vi "KE487_Test.vi"(8 "error in (no error)":errorcluster, 11 "KE487 in":refnum<class "KE487.lvclass">) -> (0 "error out":errorcluster, 3 "KE487 out":refnum<class "KE487.lvclass">)   [LabVIEW 2013, in "KE487.lvclass"]
uses:
  KE487.lvclass
  <vilib>/Platform/TimedLoop/XDataNode/timing_clust.ctl
  <vilib>/Platform/TimedLoop/XDataNode/nitl_modes.ctl
  <vilib>/Platform/TimedLoop/XDataNode/wakeup.ctl
  InstrumentSetup.vi
  <vilib>/platform/TimedLoop/XDataNode/XDataNode.xnode
  <vilib>/Platform/TimedLoop/XDataNode/XDNodeRunTimeDep.lvlib
  InstrControl.lvclass
panel:
  out "Current [nA]":dbl
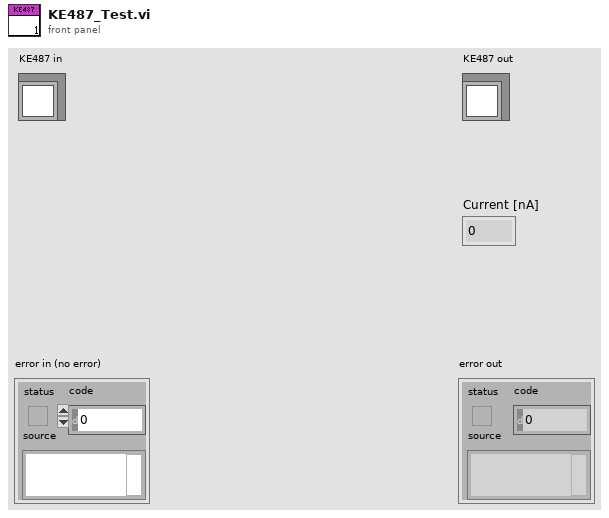
[diagram p1: front panel]
types:
  T1 = cluster{"KE 2410":cluster{"Instrument name":string, "address":refnum<visa-resource-name>, "Instrument type":u16}, "KE 6517":cluster{"Instrument name":string, "address":refnum<visa-resource-name>, "Instrument type":u16}, "KE 487":cluster{"Instrument name":string, "address":refnum<visa-resource-name>, "Instrument type":u16}, "KE 236":cluster{"Instrument name":string, "address":refnum<visa-resource-name>, "Instrument type":u16}, "WK 6440B":cluster{"Instrument name":string, "address":refnum<visa-resource-name>, "Instrument type":u16}, "WK 6425":cluster{"Instrument name":string, "address":refnum<visa-resource-name>, "Instrument type":u16}, "Pickering Matrix":cluster{"Instrument name":string, "address":refnum<visa-resource-name>, "Instrument type":u16}, "KE 2000":cluster{"Instrument name":string, "address":refnum<visa-resource-name>, "Instrument type":u16}, "KE3706A Switching":cluster{"Instrument name":string, "address":refnum<visa-resource-name>, "Instrument type":u16}}
  T2 = cluster{"Compliance":u16, "Range:":u16, "KE487":refnum<class "KE487.lvclass">}
  T3 = typedef "XDNodeRunTimeDep.lvlib/timing_clust.ctl" = cluster{"Expected End [f-1]":u64, "Actual End [f-1]":u64, "Finished Late? [f-1]":bool, "Expected End [i-1]":u64, "Actual End [i-1]":u64, "Finished Late? [i-1]":bool, "Expected Start [i]":u64, "Actual Start [i]":u64, "Expected Start [f]":u64, "Actual Start [f]":u64, "Source Name":string, "Structure Name":string, "Period":i64, "Deadline":i64, "Offset":i64, "Start":i64, "Priority":i32, "Timeout":i32, "Mode":T4, "Wakeup Reason":T5, "Error":errorcluster, "Source Type":string, "Secondary Source Type":string, "Global End Time":u64, "Global Start Time":u64, "Frame Duration":u64, "Iteration Duration":u64, "Assigned CPU":i32, "I/O Scan Engine Mode":u32}
  T4 = typedef "XDNodeRunTimeDep.lvlib/nitl_modes.ctl" = enum32{"No Change", "Process missed periods, maintain original phase", "Discard missed periods, maintain original phase", "Process missed periods, ignore original phase", "Discard missed periods, ignore original phase"}
  T5 = typedef "XDNodeRunTimeDep.lvlib/wakeup.ctl" = enum32{"Normal", "Aborted", "Asynchronous wakeup", "Timing source error", "Timed loop error", "Timeout"}
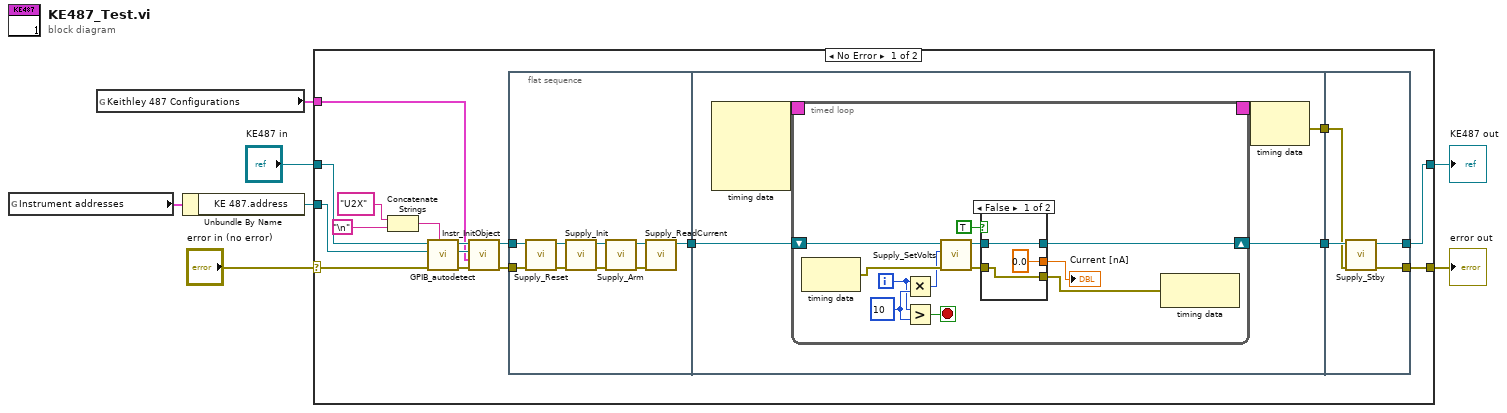
[diagram p0: block diagram]
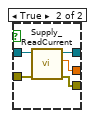
[diagram p2: hidden frame]
diagram:
  n1 = global read "InstrumentSetup.vi" "Instrument addresses"() -> (w3:T1)
  n2 = global read "InstrumentSetup.vi" "Keithley 487 Configurations"() -> (w1:T2)
  n3 = Unbundle By Name(w3) -> ("KE 487.address"=w2:refnum<visa-resource-name>)
  n4 = case shown="No Error" "error in (no error)" {
    selector: "error in (no error)" -> [w13 w72]
    tunnel: [w19 w72] -> w6
    tunnel: [w18 w71] -> w4
    tunnel: "KE487 in" -> [w17 w71]
    tunnel: w2 -> [w15 _]
    tunnel: w1 -> [w11 _]
    frame No Error {
      n5 = Concatenate Strings("U2X" ("regular expression"), "\n") -> (w8:string)
      n6 = call-dynamic "GPIB_autodetect.vi"("ID command"=w8, "error in (no error)"=w13, "Instrument address in"=w15, "InstrControl in"=w17) -> ("error out"=w12:errorcluster, "Instrument address out"=w14:refnum<visa-resource-name>, "InstrControl out"=w16:refnum<class "KE487.lvclass">)  [unwired: 5 in]
      n7 = call-dynamic "Instr_InitObject.vi"("error in (no error)"=w12, "Instrument Configuration"=w11, "Instrument address"=w14, "KE487 in"=w16) -> ("error out"=w21:errorcluster, "KE487 out"=w20:refnum<class "KE487.lvclass">)  [unwired: 6 in]
      n8 = flat-sequence {
        tunnel: w21 -> [w28]
        tunnel: w20 -> [w27]
        tunnel: [w25] -> w24
        tunnel: w24 -> [w38]
        tunnel: [w37] -> w23
        tunnel: [w34] -> w22
        tunnel: [w68] -> w19
        tunnel: w23 -> [w69]
        tunnel: w22 -> [w70]
        tunnel: [w67] -> w18
        frame #0 {
          n9 = call-dynamic "Supply_Reset.vi"("error in (no error)"=w28, "SupplyControl in"=w27) -> ("error out"=w32:errorcluster, "SupplyControl out"=w26:refnum<class "KE487.lvclass">)  [unwired: 8 in]
          n10 = call-dynamic "Supply_Init.vi"("error in (no error)"=w32, "SupplyControl in"=w26) -> ("error out"=w31:errorcluster, "SupplyControl out"=w33:refnum<class "KE487.lvclass">)  [unwired: 8 in]
          n11 = call-dynamic "Supply_Arm.vi"("error in (no error)"=w31, "SupplyControl in"=w33) -> ("error out"=w29:errorcluster, "SupplyControl out"=w30:refnum<class "KE487.lvclass">)  [unwired: 8 in]
          n12 = call-dynamic "Supply_ReadCurrent.vi"("error in (no error)"=w29, "SupplyControl in"=w30) -> ("SupplyControl out"=w25:refnum<class "KE487.lvclass">)  [unwired: 7 in, 2 out]
        }
        frame #1 {
          n13 = node-c288() -> (w36:T3)  [unwired: 4 in]
          n14 = timed-loop {
            timing: w36 -> [_]
            timing-out: [_] -> w35
            shift-right: [w42] -> w34
            shift-left: w38 -> [w48]
            i -> [w46]
            stop <- w45 stop-if-true
            w47 = 10
            n15 = node-c288() -> (w50:errorcluster)  [unwired: 1 in]
            n16 = Multiply(x=w46, y=w47) -> (x*y=w49:i32)
            n17 = Greater?(x=w46, y=w47) -> (0:w45:bool)
            n18 = call-dynamic "Supply_SetVolts.vi"("error in (no error)"=w50, "Volts IN [V]"=w49, "KE487 in"=w48) -> ("error out"=w44:errorcluster, "KE487 out"=w43:refnum<class "KE487.lvclass">)  [unwired: 6 in, 1 out]
            n19 = case shown="False" TRUE {
              tunnel: w44 -> [w53 w58]
              tunnel: w43 -> [w52 w57]
              tunnel: [w52 w56] -> w42
              tunnel: [w53 w55] -> w41
              tunnel: [0.0 w54] -> w39
              frame False {
              }
              frame True {
                n20 = call-dynamic "Supply_ReadCurrent.vi"("error in (no error)"=w58, "SupplyControl in"=w57) -> ("error out"=w55:errorcluster, "Current in nA"=w54:dbl, "SupplyControl out"=w56:refnum<class "KE487.lvclass">)  [unwired: 7 in]
              }
            }
            "Current [nA]" <- w39
            n21 = node-c288(w41) -> ()  [unwired: 1 out]
          }
          n22 = node-c288(w35) -> (w37:errorcluster)
        }
        frame #2 {
          n23 = call-dynamic "Supply_Stby.vi"("error in (no error)"=w69, "SupplyControl in"=w70) -> ("error out"=w68:errorcluster, "SupplyControl out"=w67:refnum<class "KE487.lvclass">)  [unwired: 8 in]
        }
      }
    }
    frame Error {
    }
  }
  "error out" <- w6
  "KE487 out" <- w4
